vi "Read wireRef.vi"(8 "error in (no error)":errorcluster, 11 "Wire in":refnum<class "Wire.lvclass">) -> (0 "error out":errorcluster, 2 "wireRef":refnum<vi>, 3 "Wire out":refnum<class "Wire.lvclass">)   [LabVIEW 2023, in "TLC_Scripto.lvlib" / "Wire.lvclass"]
uses:
  Wire.lvclass
  Wire.lvclass/Wire.ctl
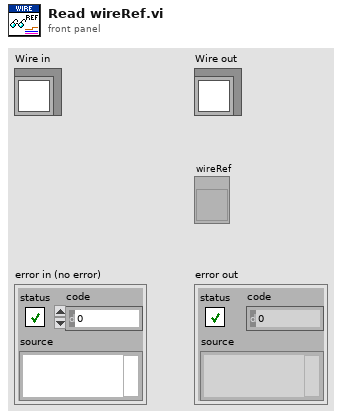
[diagram p1: front panel]
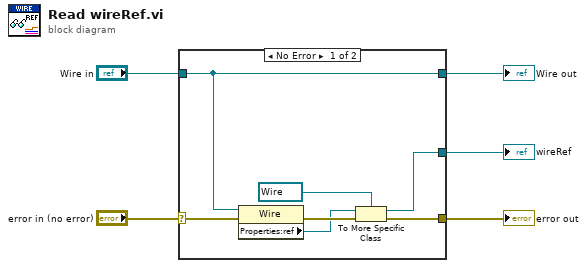
[diagram p0: block diagram]
diagram:
  n1 = case shown="No Error" "error in (no error)" {
    selector: "error in (no error)" -> [w9 w14]
    tunnel: [w8 w14] -> w4
    tunnel: [w10 w13] -> w2
    tunnel: "Wire in" -> [w10 w13]
    tunnel: [w6 _] -> w1
    frame No Error {
      n2 = property class="Wire"(reference=w10, error in=w9) -> (error out=w12:errorcluster, "Properties:ref"=w11:refnum<vi>)  [unwired: 1 out]
      n3 = To More Specific Class(target class=refnum<vi> refnum ("type"), reference=w11, error in=w12) -> (specific class reference=w6:refnum<vi>, error out=w8:errorcluster)
    }
    frame Error {
    }
  }
  "error out" <- w4
  "Wire out" <- w2
  "wireRef" <- w1
